vi "Create Step Type Menu Item.vi"(9 "Group":string, 10 "Display Name":string, 11 "Step Type":string) -> (3 "Step Type Menu Item":refnum<class "StepTypeMenuItem.lvclass">)   [LabVIEW 2020, in "TSnax UI.lvlib" / "StepTypeMenuItem.lvclass"]
uses:
  StepTypeMenuItem.lvclass
  StepTypeMenuItem.lvclass/StepTypeMenuItem.ctl
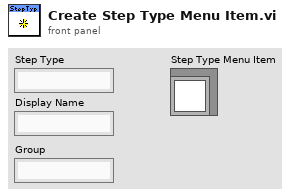
[diagram p1: front panel]
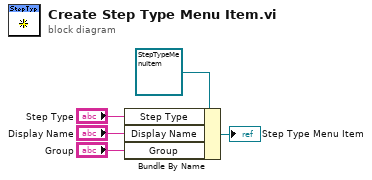
[diagram p0: block diagram]
diagram:
  n1 = Bundle By Name(cluster=refnum<class "StepTypeMenuItem.lvclass"> refnum ("TSnax UI.lvlib:StepTypeMenuItem.lvclass"), "Step Type"="Step Type", "Display Name"="Display Name", "Group"="Group") -> (→"Step Type Menu Item":refnum<class "StepTypeMenuItem.lvclass">)
